vi "Testbench for FPGA Read compass.vi"() -> ()   [LabVIEW 2011]
doc: "Simple demonstration of digital compass through cRIO. Outputs our heading on a compass.\nTo run it, you first need to run WriteToFIFO through the FPGA target (don't try running it from the folder it's in!).\nReads the data from the FPGA, passes it through and turns it into heading.\nTested with the actual sensor - it's a bit laggy, but works.\n-Elizabeth Mahon"
panel:
  out "Gauge":dbl(knob) scale=0.0..360.0
  in  "stop":bool
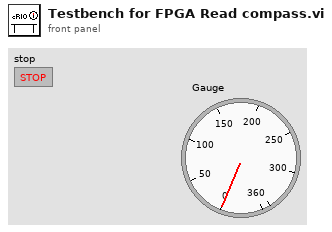
[diagram p1: front panel]
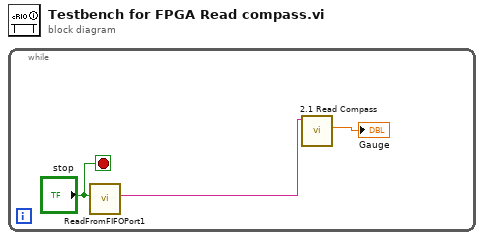
[diagram p0: block diagram]
diagram:
  n1 = while {
    stop <- "stop" stop-if-true
    n2 = call "ReadFromFIFOPort1.vi"("stop"="stop") -> ("This is what I told you!"=w1:string)  [unwired: 10 in]
    n3 = call "2.1 Read Compass.vi"("Reads a string\nfrom FPGA"=w1) -> ("heading"=→"Gauge":dbl)  [unwired: 8 in, 2 out]
  }
